vi "VMO.vi"(0 "System no.":i32=1 min=1 max=4 step=1, 2 "Axes to command":string[](array[string]), 3 "Position values":dbl[](array[numeric]) format="%.6f", 4 "No.of digits":i16=4, 5 "error in":errorcluster) -> (14 "Move possible":bool, 19 "error out":errorcluster)   [LabVIEW 2020]
doc: "Virtual movement. Indicates whether a move to the specified position is possible or not. Stage will not be moved. is the number of digits after the decimal point in the position value(s) that will be sent.\n\nC-887, F-206, M-8X0: For GCS syntax version = GCS 1.0 (check with CSV?.vi. If CSV?.vi is not supported, syntax version is GCS 1.0), VI sends command VMO. For GCS 2.0 and higher, VI sends command VMO? instead."
uses:
  Syntax.ctl
  Global1.vi
panel:
  # "Virtual movement. Indicates whether a move to the specified\nposition is possible or not. Stage will NOT be moved."
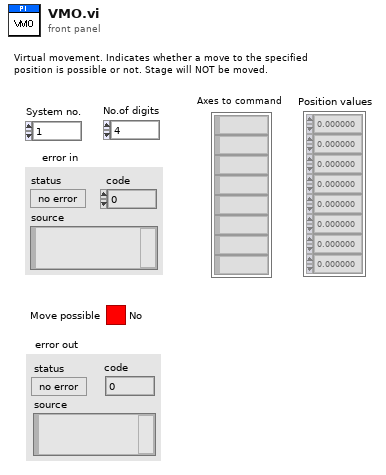
[diagram p1: front panel]
types:
  T1 = typedef "Syntax.ctl" = enum16{"GCS 1.0", "GCS 2.0", "GCS 3.0"}
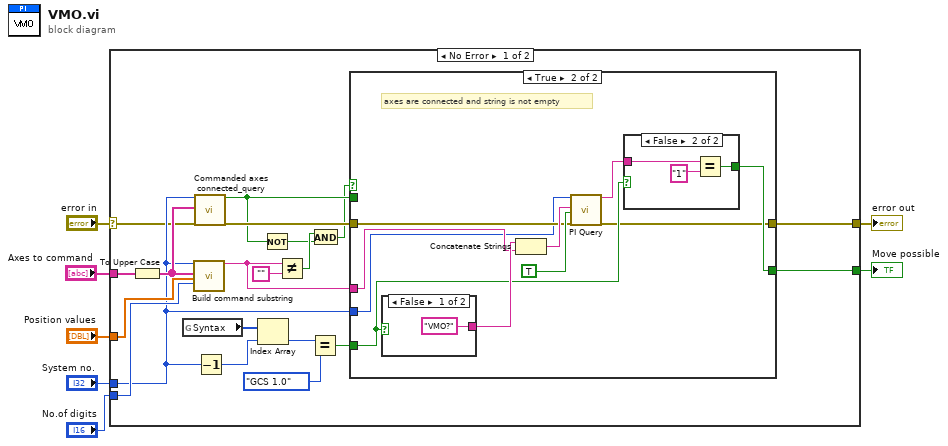
[diagram p0: block diagram]
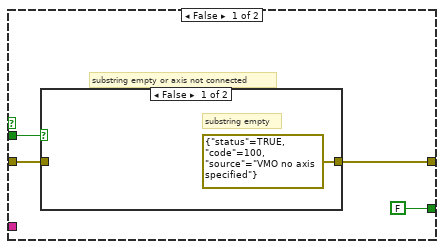
[diagram p2: hidden frame]
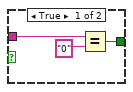
[diagram p4: hidden frame]
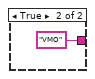
[diagram p5: hidden frame]
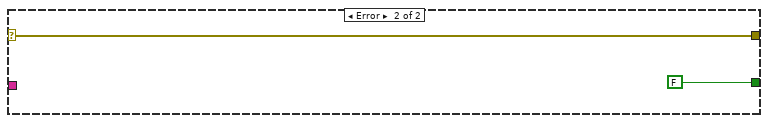
[diagram p6: hidden frame]
diagram:
  n1 = case shown="No Error" "error in" {
    selector: "error in" -> [w9 w52]
    tunnel: [w27 w52] -> w7
    tunnel: "Position values" -> [w24 _]
    tunnel: "No.of digits" -> [w23 _]
    tunnel: "System no." -> [w11 _]
    tunnel: [w17 FALSE] -> w3
    tunnel: "Axes to command" -> [w16 _]
    frame No Error {
      n2 = To Upper Case(1:w16) -> (0:w15:string[])
      n3 = global read "Global1.vi" "Syntax"() -> (w14:T1[])
      n4 = call "Build command substring.vi"("System no."=w11, "Affected axes"=w15, "Parameters"=w24, "No. of digits"=w23) -> ("Command substring"=w25:string)  [unwired: 3 in, 12 out]
      n5 = call "Commanded axes connected_query.vi"("System no."=w11, "Commanded axes"=w15, "error in"=w9) -> ("Controller error"=w20:bool, "error out"=w22:errorcluster)  [unwired: 1 in, 14 out]
      n6 = Decrement(x=w11) -> (x-1=w13:i32)
      n7 = Index Array(array=w14, index=w13) -> (element=w12:T1)
      n8 = Not(x=w20) -> (.not. x?=w19:bool)
      n9 = Not Equal?(x=w25, y="") -> (x != y?=w21:bool)
      n10 = Equal?(x=w12, y=Syntax."GCS 1.0") -> (x = y?=w10:bool)
      n11 = And(x=w21, y=w19) -> (x .and. y?=w18:bool)
      n12 = case shown="True" w18 {
        tunnel: w25 -> [_ w42]
        tunnel: [w31 w35] -> w27
        tunnel: w22 -> [w29 w39]
        tunnel: w20 -> [w30 _]
        tunnel: w11 -> [_ w38]
        tunnel: [FALSE w37] -> w17
        tunnel: w10 -> [_ w36]
        frame False {
          # "substring empty or axis not connected"
          n13 = case shown="False" w30 {
            tunnel: [errorcluster {"status"=TRUE, "code"=100, "source"="VMO no axis specified"} ("error out") w33] -> w31
            tunnel: w29 -> [_ w33]
            frame False {
              # "substring empty"
            }
            frame True {
              # "commanded axis not connected"
            }
          }
        }
        frame True {
          # "axes are connected and string is not empty"
          n14 = case shown="False" w36 {
            tunnel: ["VMO?" "VMO"] -> w43
            frame False {
            }
            frame True {
            }
          }
          n15 = Concatenate Strings(w43, w42) -> (w40:string)
          n16 = call "PI Query.vi"("System no."=w38, "String to send"=w40, "Attach termination char.?"=TRUE ("Attach Linefeed?"), "error in"=w39) -> ("String read"=w34:string, "error out"=w35:errorcluster)  [unwired: 3 in, 11 out]
          n17 = case shown="False" w36 {
            tunnel: w34 -> [w46 w49]
            tunnel: [w45 w48] -> w37
            frame True {
              n18 = Equal?(x=w46, y="0") -> (x = y?=w45:bool)
            }
            frame False {
              n19 = Equal?(x=w49, y="1") -> (x = y?=w48:bool)
            }
          }
        }
      }
    }
    frame Error {
    }
  }
  "error out" <- w7
  "Move possible" <- w3
